vi "VerifyWaveform.vi"(11 "Waveform":waveform(dbl)) -> (3 "Has Expected Value":bool)   [LabVIEW 2011]
panel:
  in  "CompareAgainstThis":waveform(dbl)={"t0"=timestamp(0 s since 1904-01-01), "dt"=0.001, "Y"=[0.5414953574552093, 1.6388780659426414, 1.7497283276545341, 1.1384679242558564, 0.9463298636900555, 1.5477997152634007, 1.3340162248639196, 1.4802927881619565, 1.5694605908778911, 2.401485637581769, 1.9883632292450393, 2.8458497455664933, 1.985583236160648, 1.974353500161004, 2.6423925169254456, 2.4575342651964993, 2.4347068127244933, 3.004237254860115, 2.352645310529958, 2.4054332773779654, 3.3984898938969827, 3.1120696495056404, 2.4368849024513546, 2.5148865251566663, 2.821140835820644, 3.5233678189543025, 3.2700361838556136, 2.9225248376391773, 3.312790094869275, 3.0605207930320866, 2.3691592744031675, 2.7263458102040037, 2.8499493582610325, 2.3080172042008376, 2.950858801928303, 2.5648100315584186, 2.592402775724249, 2.142341854518845, 2.1926296223782495, 2.601082504269755, 2.5284365166407055, 2.4302228059170052, 1.3740454717879493, 1.3296536389514926, 2.0299227198149215, 2.0882200421451045, 1.2632578138176884, 1.5569259738640602, 0.9213172934051927, 1.6626458201575987, 0.559712587995601, 0.665849635545508, 0.7557759935709658, 0.33743796301234996, 0.2792081936279984, -0.17410243448845902, 0.6042491019769984, 0.15335877961801692, 0.26634930444981425, -0.5366760054863771, -0.6184571839480917, -0.7907989217295364, -0.1470498937869107, -0.23356323972390602, -0.5237685796348657, -1.1497555570049447, -1.1697783355446882, -0.7450493517392278, -0.31599656859320613, -0.921614147205145, -0.7482234695080388, -1.342706695401521, -1.5329523342843832, -1.3946572950654208, -0.5885005084790296, -1.180953321964905, -0.9000215445196414, -1.229682263865325, -0.9232931284406605, -0.9532185724798816, -0.3875989384031755, -0.5922091965434321, -0.5754544786294116, -0.2567368326137988, -0.19025045265598528, -0.9600864552518067, -0.10129419384882721, -0.3971806680502059, -0.1760237288932313, 0.3750398520477397, 0.21710921088274504, -0.3109622957739306, -0.09933080312465892, 0.16321088986745536, 0.7094569577585599, 1.0578965269007958, 0.03661422048334717, 0.5861028554571415, 1.4042849916784088, 0.6991105993713287], "attributes"=variant("NI_ChannelName"=variant(string "Sine with Uniform Noise"), "NI_ExpIsRelativeTime"=variant(bool TRUE), "NI_ExpStartTimeStamp"=variant(timestamp timestamp(3325237824.8125 s since 1904-01-01)), "NI_ExpTimeStamp"=variant(timestamp timestamp(3325237824.8125 s since 1904-01-01)), "NI_ExpXDimension"=variant(string "t"))}
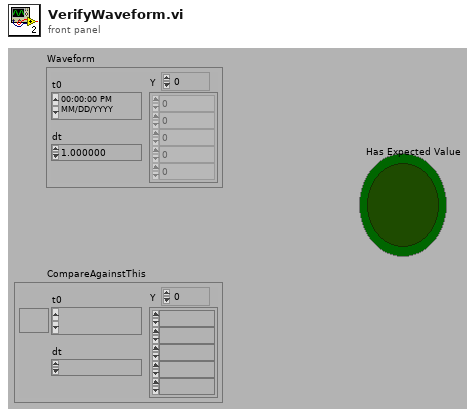
[diagram p1: front panel]
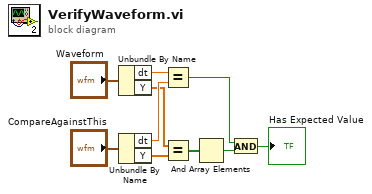
[diagram p0: block diagram]
diagram:
  n1 = Unbundle By Name("Waveform") -> ("dt"=w8:dbl, "Y"=w6:dbl[])
  n2 = Unbundle By Name("CompareAgainstThis") -> ("dt"=w7:dbl, "Y"=w5:dbl[])
  n3 = Equal?(x=w8, y=w7) -> (x = y?=w3:bool)
  n4 = Equal?(x=w6, y=w5) -> (x = y?=w4:bool[])
  n5 = And Array Elements(Boolean array=w4) -> (logical AND=w2:bool)
  n6 = And(x=w3, y=w2) -> (x .and. y?=→"Has Expected Value":bool)
